vi "Calculate criteria.vi"(5 "Criteria":T1, 7 "Sequence step started":timestamp, 9 "Operator presse OK":bool, 13 "User input 1":dbl) -> (6 "Continue":bool, 8 "Unknown":bool, 10 "Show opperator aproval  button":bool)   [LabVIEW 2011]
uses:
  Single criteria cluster.ctl
  Criteria types.ctl
  Measurments Handling/Action Analog Handler.ctl
  Measurments Handling/Status Digitalish.ctl
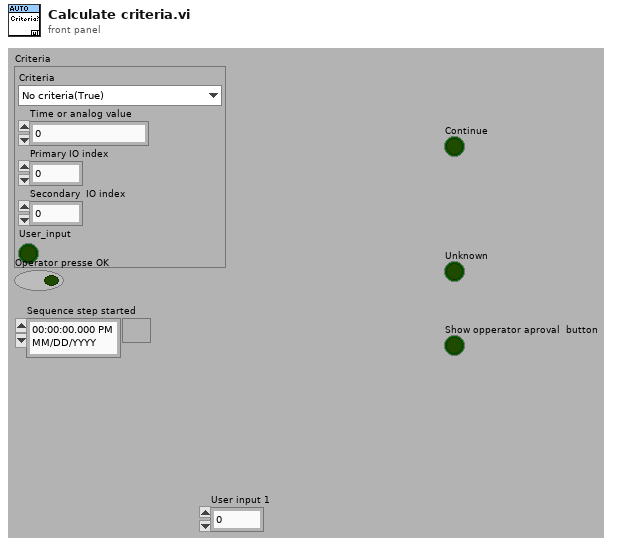
[diagram p1: front panel]
types:
  T1 = typedef "Single criteria cluster.ctl" = cluster{"Criteria":T2, "Time or analog value":dbl, "Primary IO index":i32, "Secondary  IO index":i32, "User_input":bool}
  T2 = typedef "Criteria types.ctl" = enum16{"No criteria(True)", "Time(s)", "Analog IO over", "Analog IO over or equal", "Analog IO under", "Analog IO under or equal", "Analog IO 1 minus Analog IO 2 over", "Digital IO True", "Digital IO False", "Operator approval"}
  T3 = typedef "Action Analog Handler.ctl" = enum16{"GET value", "GET Single Frequenzy", "GET All Values", "GET Waveform", "Get Numb Var", "SET Value", "START Buffer", "REG Variable", "BUF size(total antal sekund)", "PULS", "Get a Value at time", "Set initial waveform"}
  T4 = typedef "Status Digitalish.ctl" = enum16{"NA", "False", "True"}
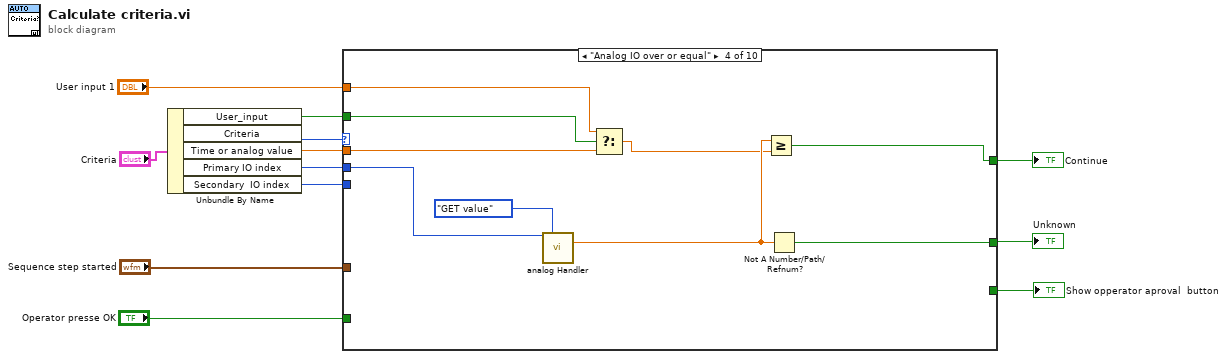
[diagram p0: block diagram]
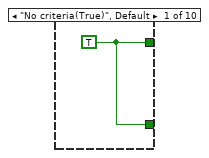
[diagram p2: hidden frame]
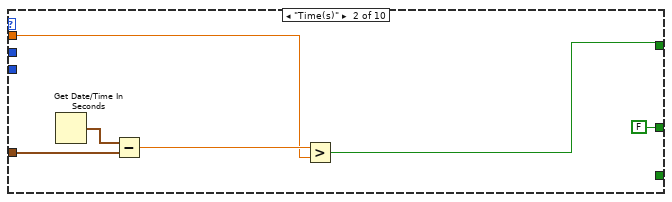
[diagram p3: hidden frame]
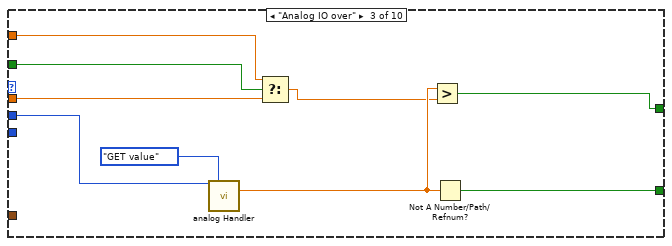
[diagram p4: hidden frame]
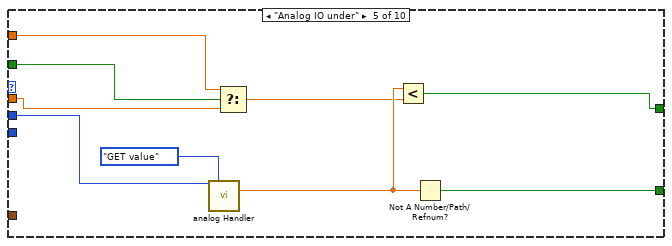
[diagram p5: hidden frame]
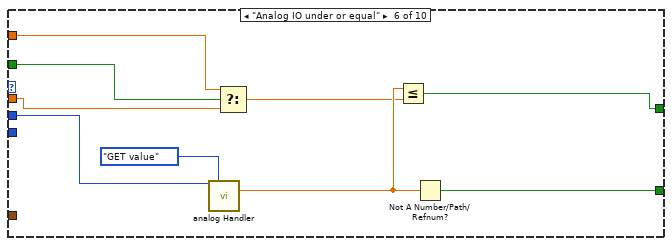
[diagram p6: hidden frame]
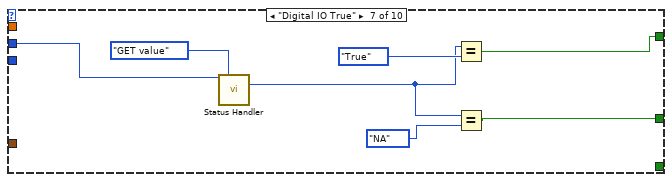
[diagram p7: hidden frame]
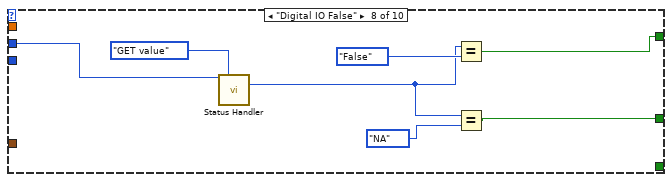
[diagram p8: hidden frame]
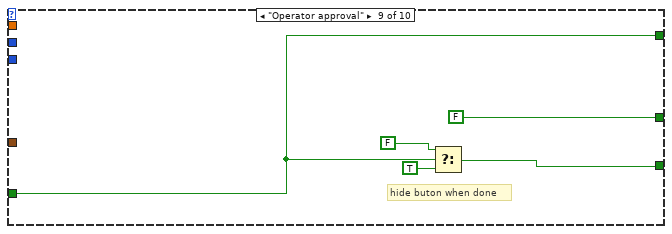
[diagram p9: hidden frame]
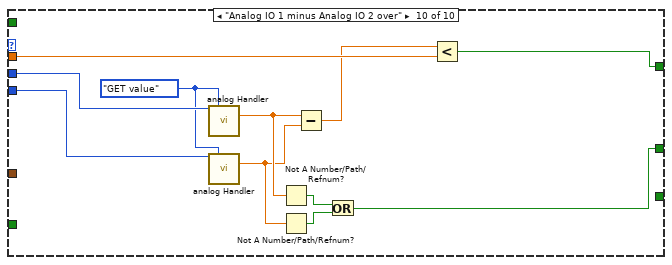
[diagram p10: hidden frame]
diagram:
  n1 = Unbundle By Name("Criteria") -> ("User_input"=w2:bool, "Criteria"=w11:T2, "Time or analog value"=w10:dbl, "Primary IO index"=w9:i32, "Secondary  IO index"=w8:i32)
  n2 = case shown="\"Analog IO over or equal\"" w11 {
    tunnel: w10 -> [_ w16 w21 w30 w39 w48 _ _ _ w84]
    tunnel: w9 -> [_ _ w27 w36 w45 w54 w61 w68 _ w85]
    tunnel: w8 -> [_ _ _ _ _ _ _ _ _ w81]
    tunnel: "Sequence step started" -> [_ w18 _ _ _ _ _ _ _ _]
    tunnel: [w13 w15 w26 w35 w44 w53 w56 w63 w72 w83] -> w6
    tunnel: [w13 FALSE w24 w33 w42 w51 w60 w67 FALSE w75] -> w5
    tunnel: "Operator presse OK" -> [_ _ _ _ _ _ _ _ w72 _]
    tunnel: [_ _ _ _ _ _ _ _ w73 _] -> w3
    tunnel: w2 -> [_ _ w22 w31 w41 w50 _ _ _ _]
    tunnel: "User input 1" -> [_ _ w20 w29 w40 w49 _ _ _ _]
    frame "No criteria(True)", Default {
      w13 = TRUE
    }
    frame "Time(s)" {
      n3 = Get Date/Time In Seconds() -> (seconds since 1Jan1904=w19:timestamp)
      n4 = Subtract(x=w19, y=w18) -> (x-y=w17:dbl)
      n5 = Greater?(x=w17, y=w16) -> (0:w15:bool)
    }
    frame "Analog IO over" {
      n6 = call "analog Handler.vi"("Variable Index"=w27, "Action"=Action_Analog_Handler."GET value") -> ("Value out"=w25:dbl)  [unwired: 8 in, 5 out]
      n7 = Select(t=w20, s=w22, f=w21) -> (s? t:f=w23:dbl)
      n8 = Greater?(x=w25, y=w23) -> (0:w26:bool)
      n9 = Not A Number/Path/Refnum?(number/path/refnum=w25) -> (NaN/Path/Refnum?=w24:bool)
    }
    frame "Analog IO over or equal" {
      n10 = call "analog Handler.vi"("Variable Index"=w36, "Action"=Action_Analog_Handler."GET value") -> ("Value out"=w34:dbl)  [unwired: 8 in, 5 out]
      n11 = Select(t=w29, s=w31, f=w30) -> (s? t:f=w32:dbl)
      n12 = Greater Or Equal?(x=w34, y=w32) -> (x >= y?=w35:bool)
      n13 = Not A Number/Path/Refnum?(number/path/refnum=w34) -> (NaN/Path/Refnum?=w33:bool)
    }
    frame "Analog IO under" {
      n14 = call "analog Handler.vi"("Variable Index"=w45, "Action"=Action_Analog_Handler."GET value") -> ("Value out"=w43:dbl)  [unwired: 8 in, 5 out]
      n15 = Select(t=w40, s=w41, f=w39) -> (s? t:f=w38:dbl)
      n16 = Less?(x=w43, y=w38) -> (x < y?=w44:bool)
      n17 = Not A Number/Path/Refnum?(number/path/refnum=w43) -> (NaN/Path/Refnum?=w42:bool)
    }
    frame "Analog IO under or equal" {
      n18 = call "analog Handler.vi"("Variable Index"=w54, "Action"=Action_Analog_Handler."GET value") -> ("Value out"=w52:dbl)  [unwired: 8 in, 5 out]
      n19 = Select(t=w49, s=w50, f=w48) -> (s? t:f=w47:dbl)
      n20 = Less Or Equal?(x=w52, y=w47) -> (x <= y?=w53:bool)
      n21 = Not A Number/Path/Refnum?(number/path/refnum=w52) -> (NaN/Path/Refnum?=w51:bool)
    }
    frame "Digital IO True" {
      n22 = call "Status Handler.vi"("Variable Index"=w61, "Action"=Action_Analog_Handler."GET value") -> ("Value out"=w57:T4)  [unwired: 9 in, 4 out]
      n23 = Equal?(x=w57, y=Status_Digitalish."True" ("Value out")) -> (x = y?=w56:bool)
      n24 = Equal?(x=w57, y=Status_Digitalish."NA" ("Value out")) -> (x = y?=w60:bool)
    }
    frame "Digital IO False" {
      n25 = call "Status Handler.vi"("Variable Index"=w68, "Action"=Action_Analog_Handler."GET value") -> ("Value out"=w64:T4)  [unwired: 9 in, 4 out]
      n26 = Equal?(x=w64, y=Status_Digitalish."False" ("Value out")) -> (x = y?=w63:bool)
      n27 = Equal?(x=w64, y=Status_Digitalish."NA" ("Value out")) -> (x = y?=w67:bool)
    }
    frame "Operator approval" {
      # "hide buton when done"
      n28 = Select(t=FALSE ("Show opperator aproval  button"), s=w72, f=TRUE) -> (s? t:f=w73:bool)
    }
    frame "Analog IO 1 minus Analog IO 2 over" {
      w82 = Action_Analog_Handler."GET value" ("Action")
      n29 = call "analog Handler.vi"("Variable Index"=w85, "Action"=w82) -> ("Value out"=w79:dbl)  [unwired: 8 in, 5 out]
      n30 = call "analog Handler.vi"("Variable Index"=w81, "Action"=w82) -> ("Value out"=w78:dbl)  [unwired: 8 in, 5 out]
      n31 = Not A Number/Path/Refnum?(number/path/refnum=w79) -> (NaN/Path/Refnum?=w77:bool)
      n32 = Not A Number/Path/Refnum?(number/path/refnum=w78) -> (NaN/Path/Refnum?=w76:bool)
      n33 = Subtract(x=w79, y=w78) -> (x-y=w80:dbl)
      n34 = Or(x=w77, y=w76) -> (x .or. y?=w75:bool)
      n35 = Less?(x=w80, y=w84) -> (x < y?=w83:bool)
    }
  }
  "Continue" <- w6
  "Unknown" <- w5
  "Show opperator aproval  button" <- w3
